vi "CalculateStartupFeature.vi"(0 "current waveforms":waveform(sgl)[](array[waveform]), 5 "nameplate frequency":dbl, 7 "Full Load Amps":dbl, 9 "start trigger level [%]":dbl format="%.2p", 11 "stop trigger level [%]":dbl format="%.2p") -> (4 "startup peak amps":dbl, 6 "startup time":dbl, 10 "startup start time":timestamp)   [LabVIEW 2017, in "McsaAnalysisFunctions.lvlib"]
uses:
  <vilib>/addons/InsightCM/Utilities/Analysis/MCSA/McsaAnalysisFunctions.lvlib
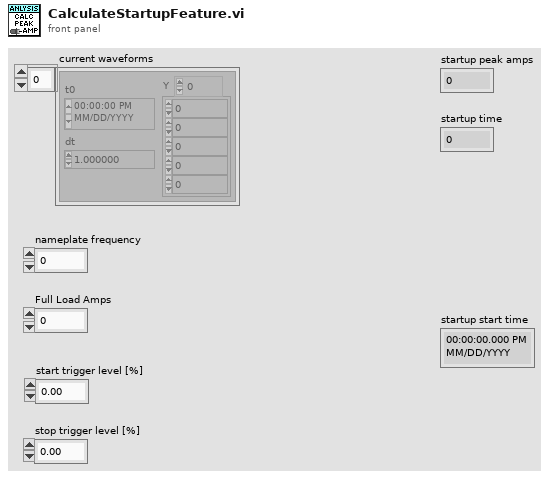
[diagram p1: front panel]
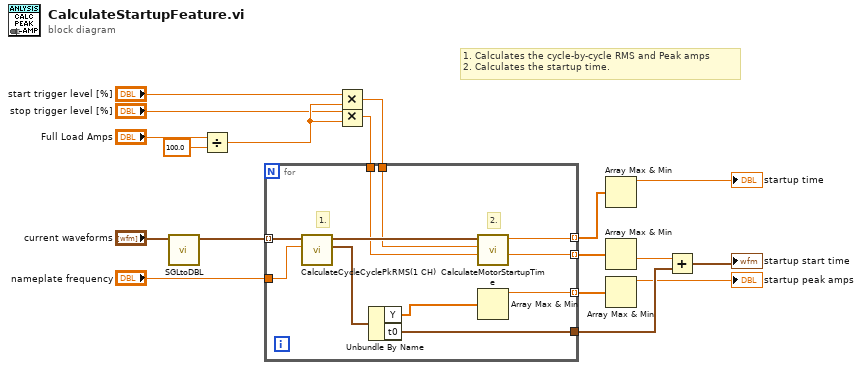
[diagram p0: block diagram]
diagram:
  # "1. Calculates the cycle-by-cycle RMS and Peak amps\n2. Calculates the startup time."
  n1 = call <vilib>:"SGLtoDBL.vi"("SGL"="current waveforms") -> ("Double"=w3:waveform(dbl)[])  [unwired: 10 in]
  n2 = Divide(x="Full Load Amps", y=100.0) -> (x/y=w16:dbl)
  n3 = Multiply(x="start trigger level [%]", y=w16) -> (x*y=w11:dbl)
  n4 = Multiply(x="stop trigger level [%]", y=w16) -> (x*y=w12:dbl)
  n5 = for {
    tunnel: w3 -> [w29] mode=indexing
    tunnel: "nameplate frequency" -> [w28]
    tunnel: [w19] -> w17 mode=indexing
    tunnel: [w24] -> w8 mode=indexing
    tunnel: w12 -> [w23]
    tunnel: w11 -> [w22]
    tunnel: [w21] -> w7 mode=indexing
    tunnel: [w20] -> w5
    # "2."
    # "1."
    n6 = call <vilib>:"CalculateCycleCyclePkRMS(1 CH).vi"("line frequency"=w28, "waveform"=w29) -> ("peak waveform"=w26:waveform(dbl), "rms waveform"=w25:waveform(dbl))  [unwired: 7 in, 1 out]
    n7 = Unbundle By Name(w26) -> ("Y"=w27:dbl[], "t0"=w20:timestamp)
    n8 = call <vilib>:"CalculateMotorStartupTime.vi"("stop trigger level [RMS]"=w23, "start trigger level [RMS]"=w22, "waveform"=w25) -> ("startup start time"=w21:dbl, "startup time"=w24:dbl)  [unwired: 6 in, 1 out]
    n9 = Array Max & Min(array=w27) -> (max value=w19:dbl)  [unwired: 3 out]
  }
  n10 = Array Max & Min(array=w8) -> (max value=→"startup time":dbl)  [unwired: 3 out]
  n11 = Array Max & Min(array=w7) -> (min value=w6:dbl)  [unwired: 3 out]
  n12 = Array Max & Min(array=w17) -> (max value=→"startup peak amps":dbl)  [unwired: 3 out]
  n13 = Add(x=w6, y=w5) -> (x+y=→"startup start time":timestamp)
